vi "Interpolate Drive System.vi"(8 "Duration":dbl, 9 "Current Time":dbl, 10 "Start Robot Commands":T1, 11 "End Robot Commands":T1) -> (3 "Current Robot Commands":T1)   [LabVIEW 2019]
uses:
  Controls/Robot Pivot Motion Commands.ctl
  Controls/Pivot Motor Commands.ctl
  Controls/Robot Drive Mode.ctl
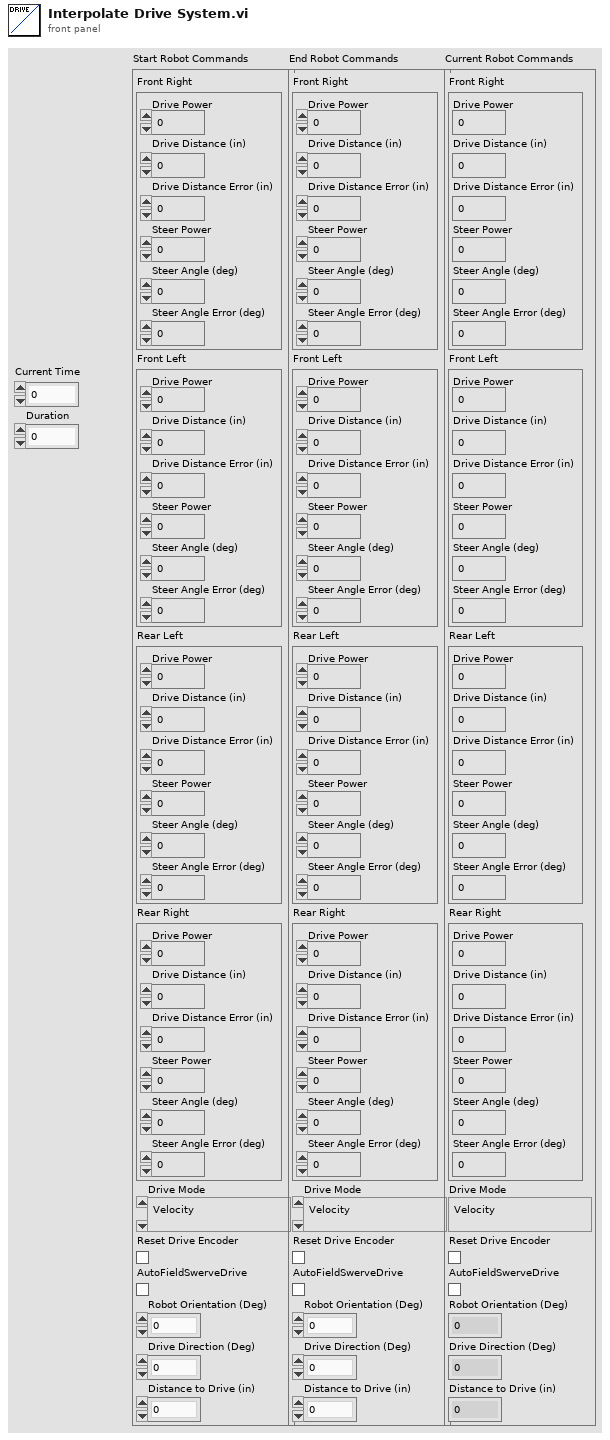
[diagram p1: front panel]
types:
  T1 = typedef "Robot Pivot Motion Commands.ctl" = cluster{"Front Right":T2, "Front Left":T2, "Rear Left":T2, "Rear Right":T2, "Drive Mode":T3, "Reset Drive Encoder":bool, "AutoFieldSwerveDrive":bool, "Robot Orientation (Deg)":dbl, "Drive Direction (Deg)":dbl, "Distance to Drive (in)":dbl}
  T2 = typedef "Pivot Motor Commands.ctl" = cluster{"Drive Power":dbl, "Drive Distance (in)":dbl, "Drive Distance Error (in)":dbl, "Steer Power":dbl, "Steer Angle (deg)":dbl, "Steer Angle Error (deg)":dbl}
  T3 = typedef "Robot Drive Mode.ctl" = enum16{"Velocity", "Distance"}
  T4 = cluster{"Current Value[0]":dbl, "Current Value[1]":dbl, "Current Value[2]":dbl, "Current Value[3]":dbl, "Current Value[4]":dbl, "Current Value[5]":dbl}
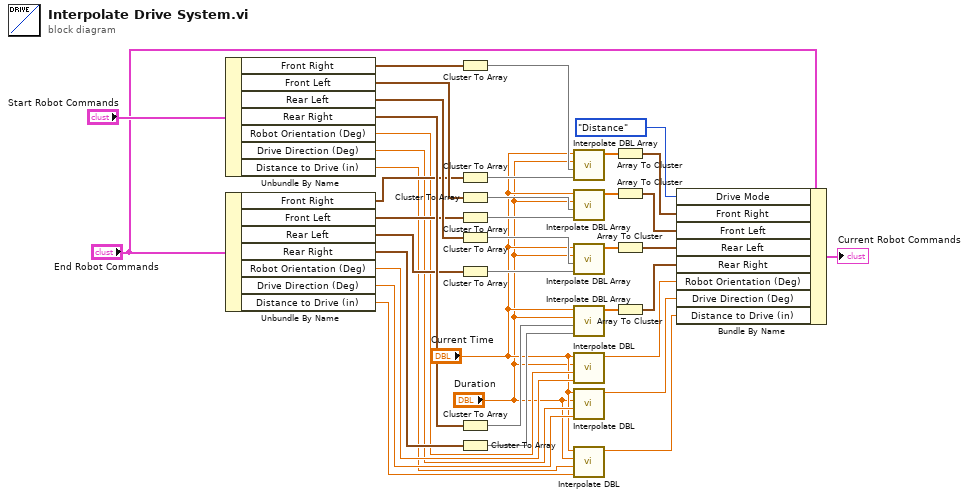
[diagram p0: block diagram]
diagram:
  n1 = Unbundle By Name("Start Robot Commands") -> ("Front Right"=w36:T2, "Front Left"=w34:T2, "Rear Left"=w31:T2, "Rear Right"=w32:T2, "Robot Orientation (Deg)"=w6:dbl, "Drive Direction (Deg)"=w7:dbl, "Distance to Drive (in)"=w8:dbl)
  n2 = Unbundle By Name("End Robot Commands") -> ("Front Right"=w21:T2, "Front Left"=w20:T2, "Rear Left"=w19:T2, "Rear Right"=w18:T2, "Robot Orientation (Deg)"=w11:dbl, "Drive Direction (Deg)"=w10:dbl, "Distance to Drive (in)"=w9:dbl)
  n3 = Cluster To Array(cluster=w36) -> (array=w35:dbl[])
  n4 = Cluster To Array(cluster=w21) -> (array=w17:dbl[])
  n5 = Cluster To Array(cluster=w34) -> (array=w33:dbl[])
  n6 = Cluster To Array(cluster=w20) -> (array=w15:dbl[])
  n7 = Cluster To Array(cluster=w31) -> (array=w30:dbl[])
  n8 = Cluster To Array(cluster=w19) -> (array=w16:dbl[])
  n9 = Cluster To Array(cluster=w32) -> (array=w29:dbl[])
  n10 = Cluster To Array(cluster=w18) -> (array=w14:dbl[])
  n11 = call "Interpolate DBL Array.vi"("Ending Value"=w17, "Starting Value"=w35, "Duration"="Duration", "Current Time"="Current Time") -> ("Current Value"=w27:dbl[])  [unwired: 7 in]
  n12 = call "Interpolate DBL Array.vi"("Ending Value"=w15, "Starting Value"=w33, "Duration"="Duration", "Current Time"="Current Time") -> ("Current Value"=w24:dbl[])  [unwired: 7 in]
  n13 = call "Interpolate DBL Array.vi"("Ending Value"=w16, "Starting Value"=w30, "Duration"="Duration", "Current Time"="Current Time") -> ("Current Value"=w25:dbl[])  [unwired: 7 in]
  n14 = call "Interpolate DBL Array.vi"("Ending Value"=w14, "Starting Value"=w29, "Duration"="Duration", "Current Time"="Current Time") -> ("Current Value"=w23:dbl[])  [unwired: 7 in]
  n15 = call "Interpolate DBL.vi"("Ending Value"=w11, "Starting Value"=w6, "Duration"="Duration", "Current Time"="Current Time") -> ("Current Value"=w1:dbl)  [unwired: 7 in]
  n16 = call "Interpolate DBL.vi"("Ending Value"=w10, "Starting Value"=w7, "Duration"="Duration", "Current Time"="Current Time") -> ("Current Value"=w2:dbl)  [unwired: 7 in]
  n17 = call "Interpolate DBL.vi"("Ending Value"=w9, "Starting Value"=w8, "Duration"="Duration", "Current Time"="Current Time") -> ("Current Value"=w3:dbl)  [unwired: 7 in]
  n18 = Array To Cluster(array=w27) -> (cluster=w26:T4)
  n19 = Array To Cluster(array=w24) -> (cluster=w12:T4)
  n20 = Array To Cluster(array=w25) -> (cluster=w13:T4)
  n21 = Array To Cluster(array=w23) -> (cluster=w22:T4)
  n22 = Bundle By Name(cluster="End Robot Commands", "Drive Mode"=Robot_Drive_Mode."Distance", "Front Right"=w26, "Front Left"=w12, "Rear Left"=w13, "Rear Right"=w22, "Robot Orientation (Deg)"=w1, "Drive Direction (Deg)"=w2, "Distance to Drive (in)"=w3) -> (→"Current Robot Commands":T1)
